vi "(Incomplete) Elliptic Integral E.vi"(2 "a":dbl=nan format="%.2f", 3 "k":dbl format="%.2f") -> (1 "E(k, a)":dbl format="%.2f")   [LabVIEW 2017, in "NI_Gmath.lvlib"]
doc: "Computes the Legendre elliptic integral of the second kind. It computes the complete elliptic integral of the second kind if you do not wire <B>a</B>."
uses:
  NI_Gmath.lvlib
  Incomplete Elliptic Integral E.vi
  Complete Elliptic Integral E.vi
panel:
  # "This VI is obsolete !!!\nYou should replace this VI in your diagram with the \nElliptic Integral of the 2nd kind VI.\n\nNOTE:   Please be aware that the new Elliptic Integral of\n             the 2nd kind VI is a polymorphic VI. If you leave \n             the a input of this obsolete VI unwired, please use \n             the Complete Elliptic Integral E instance of the \n             new Elliptic Integral of the 2nd kind VI."
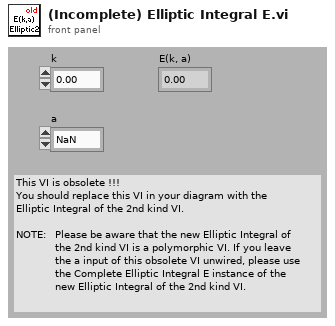
[diagram p1: front panel]
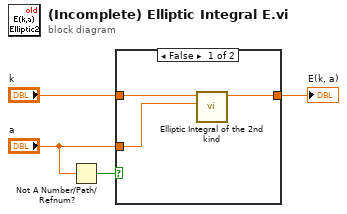
[diagram p0: block diagram]
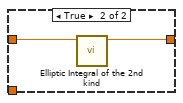
[diagram p2: hidden frame]
diagram:
  n1 = Not A Number/Path/Refnum?(number/path/refnum="a") -> (NaN/Path/Refnum?=w4:bool)
  n2 = case shown="False" w4 {
    tunnel: "k" -> [w6 w9]
    tunnel: "a" -> [w5 _]
    tunnel: [w7 w8] -> w1
    frame False {
      n3 = call-poly "Elliptic Integral of the 2nd kind.vi"("a"=w5, "k"=w6) -> ("E(k, a)"=w7:dbl)  [unwired: 9 in]
    }
    frame True {
      n4 = call-poly "Elliptic Integral of the 2nd kind.vi"("k"=w9) -> ("E(k)"=w8:dbl)  [unwired: 10 in]
    }
  }
  "E(k, a)" <- w1
